vi "intensity_weight_height.vi"() -> ()   [LabVIEW 2021]
uses:
  <vilib>/Utility/file.llb/Read Delimited Spreadsheet (string).vi
  <vilib>/Analysis/NI_AALBase.lvlib
panel:
  out "Intensity Graph":i16[][](graph)
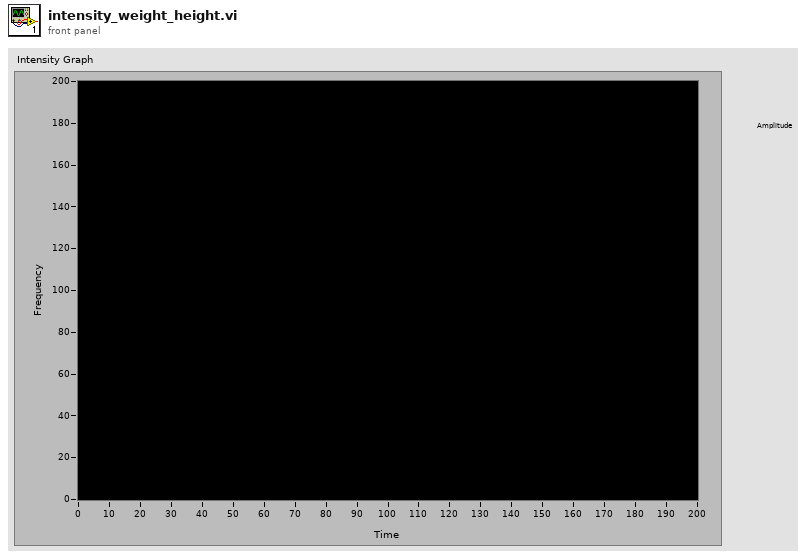
[diagram p1: front panel]
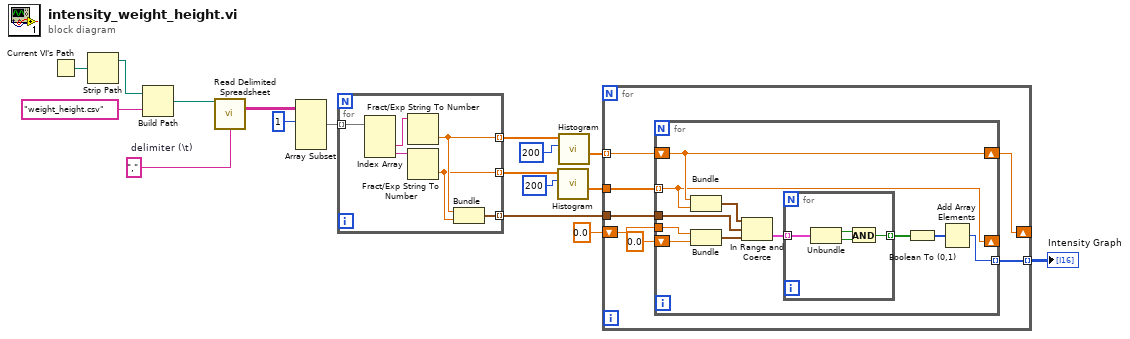
[diagram p0: block diagram]
diagram:
  w13 = ","  # delimiter (\t)
  n1 = Current VI's Path() -> (path=w17:path)
  n2 = Strip Path(path=w17) -> (stripped path=w16:path)  [unwired: 1 out]
  n3 = Build Path(base path=w16, name or relative path="weight_height.csv") -> (appended path=w14:path)
  n4 = call-poly <vilib>:"Read Delimited Spreadsheet.vi"("file path (dialog if empty)"=w14, "delimiter (\\t)"=w13) -> ("all rows"=w12:string[][])  [unwired: 8 in, 5 out]
  n5 = Array Subset(array=w12, index (row)=1 ("index")) -> (w10:string[][])  [unwired: 3 in]
  n6 = for {
    tunnel: w10 -> [w23] mode=indexing
    tunnel: [w20] -> w6 mode=indexing
    tunnel: [w19] -> w5 mode=indexing
    tunnel: [w18] -> w4 mode=indexing
    n7 = Index Array(array=w23) -> (element #2=w22:string, element #3=w21:string)  [unwired: 3 in, 1 out]
    n8 = Fract/Exp String To Number(string=w22) -> (number=w20:dbl)  [unwired: 3 in, 1 out]
    n9 = Fract/Exp String To Number(string=w21) -> (number=w19:dbl)  [unwired: 3 in, 1 out]
    n10 = Bundle(w20, w19) -> (w18:cluster{dbl, dbl})  [unwired: 1 in]
  }
  n11 = call <vilib>:"Histogram.vi"("intervals"=200, "X"=w5) -> ("X Values"=w9:dbl[])  [unwired: 6 in, 3 out]
  n12 = call <vilib>:"Histogram.vi"("intervals"=200, "X"=w6) -> ("X Values"=w8:dbl[])  [unwired: 6 in, 3 out]
  n13 = for {
    tunnel: w8 -> [w27] mode=indexing
    tunnel: w9 -> [w29]
    shift-right: [w30] -> _
    shift-left: 0.0 -> [w26]
    tunnel: w4 -> [w25]
    tunnel: [w24] -> w3 mode=indexing
    n14 = for {
      shift-right: [w38] -> w30
      shift-left: w27 -> [w38]
      shift-right: [w37] -> _
      shift-left: 0.0 -> [w40]
      tunnel: w29 -> [w37] mode=indexing
      tunnel: w26 -> [w41]
      tunnel: w25 -> [w35]
      tunnel: [w31] -> w24 mode=indexing
      n15 = Bundle(w38, w37) -> (w36:cluster{dbl, dbl})  [unwired: 1 in]
      n16 = Bundle(w41, w40) -> (w39:cluster{dbl, dbl})  [unwired: 1 in]
      n17 = In Range and Coerce(upper limit=w36, x=w35, lower limit=w39) -> (In Range?=w34:cluster{bool, bool}[])  [unwired: 1 out]
      n18 = for {
        tunnel: w34 -> [w45] mode=indexing
        tunnel: [w42] -> w33 mode=indexing
        n19 = Unbundle(w45) -> (w44:bool, w43:bool)
        n20 = And(x=w44, y=w43) -> (x .and. y?=w42:bool)
      }
      n21 = Boolean To (0,1)(Boolean=w33) -> (0, 1=w32:i16[])
      n22 = Add Array Elements(numeric array=w32) -> (sum=w31:i16)
    }
  }
  "Intensity Graph" <- w3
